vi "TIV extract element.vi"(1 "Column":i32, 2 "Row":i32, 3 "Table":string[][](table)) -> (0 "Element":dbl)   [LabVIEW 2009]
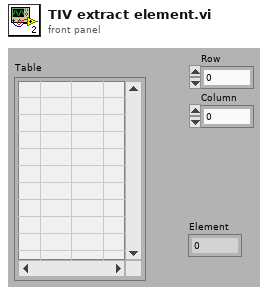
[diagram p1: front panel]
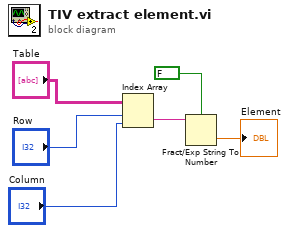
[diagram p0: block diagram]
diagram:
  n1 = Index Array(array="Table", index (row)="Row", index (col)="Column") -> (element=w3:string)
  n2 = Fract/Exp String To Number(use system decimal point (T)=FALSE, string=w3) -> (number=→"Element":dbl)  [unwired: 2 in, 1 out]
